vi "Handle Error.vi"(7 "Stop on Unhandled Error (T)":bool=TRUE, 8 "error in":errorcluster, 11 "LevyLab Instrument UI":refnum<class "LevyLab Instrument UI.lvclass">) -> (0 "handling error":errorcluster, 2 "Unhandled error":errorcluster, 3 "LevyLab Instrument UI out":refnum<class "LevyLab Instrument UI.lvclass">)   [LabVIEW 2016]
doc: "JKI State Machine Objects (SMO) 1.0.0.11\nJKI - JKI\nCopyright (c) 2016, JKIJKI State Machine Objects (SMO) 1.3.0.56\nJKI - JKI\nCopyright (c) 2017, JKI"
uses:
  LevyLab Instrument UI.lvclass
panel:
  # "For instructions on how to use the JKI State Machine Objects, examples and video tutorials, visit:\nhttp://jki.net/state-machine-objects/\n\nJKI State Machine Objects™\nhttp://jki.net/state-machine-objects/\nCopyright (C) 2005-2015, JKI <info@jki.net>\nALL RIGHTS RESERVED"
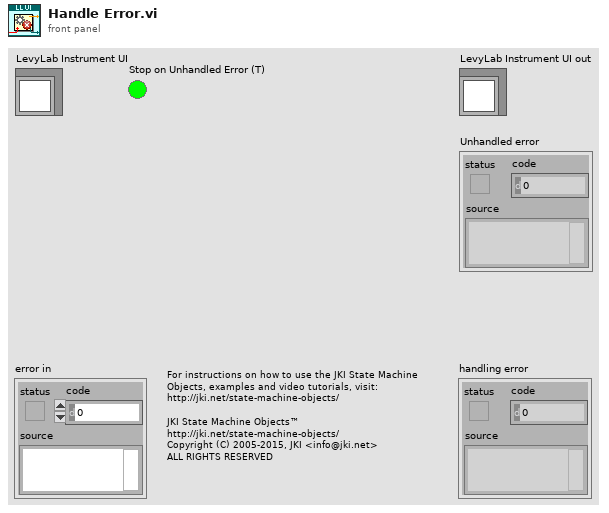
[diagram p1: front panel]
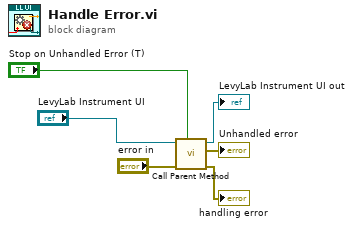
[diagram p0: block diagram]
diagram:
  n1 = call-parent "Call Parent Method"("Stop on Unhandled Error (T)"="Stop on Unhandled Error (T)", "error in"="error in", "Instrument UI"="LevyLab Instrument UI") -> ("handling error"=→"handling error":errorcluster, "Unhandled error"=→"Unhandled error":errorcluster, "Instrument UI out"=→"LevyLab Instrument UI out":refnum<class "LevyLab Instrument UI.lvclass">)  [unwired: 6 in]
